vi "fgv_viLauch.vi"(7 "Option":T1(ring), 8 "Error In":errorcluster, 10 "vi path":path, 11 "UI in":refnum<class "UI.lvclass">) -> (0 "Error Out":errorcluster, 2 "VI ref Out":refnum<vi>, 3 "UI out":refnum<class "UI.lvclass">)   [LabVIEW 2018, in "Panel.lvclass"]
uses:
  Panel.lvclass
  User Interface/UI.lvclass
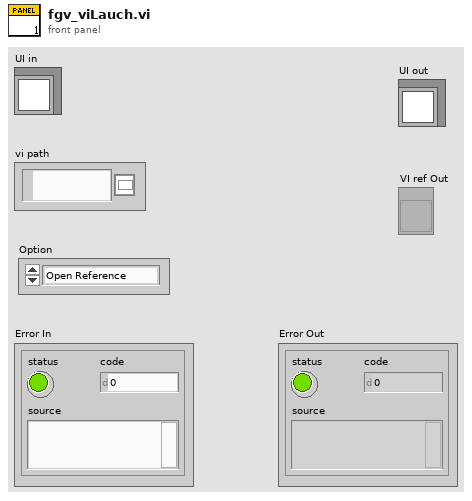
[diagram p1: front panel]
types:
  T1 = enum16{"Open Reference", "Launch VI", "Get VI Outputs"}
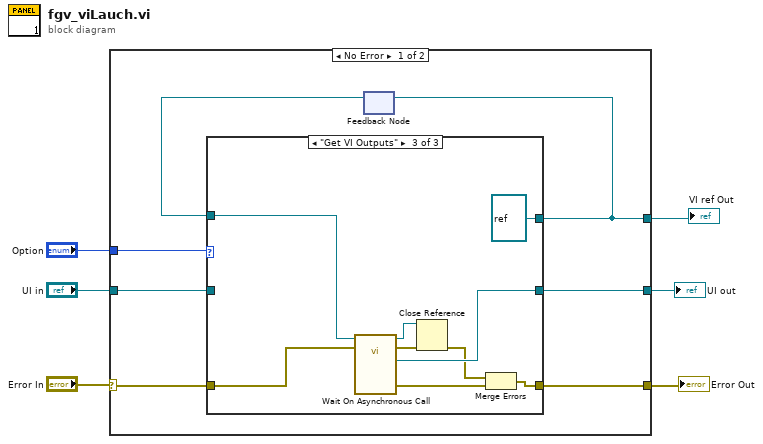
[diagram p0: block diagram]
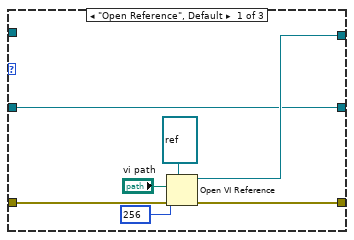
[diagram p2: hidden frame]
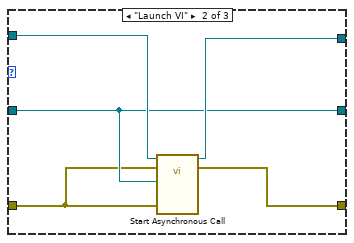
[diagram p3: hidden frame]
diagram:
  n1 = case shown="No Error" "Error In" {
    selector: "Error In" -> [w13 w35]
    tunnel: [w12 w35] -> w5
    tunnel: "Option" -> [w11 _]
    tunnel: [w9 w36] -> w3
    tunnel: "UI in" -> [w8 w36]
    tunnel: [w7 _] -> w1
    frame No Error {
      n2 = feedback #1() -> (w10:refnum<vi>)  [unwired: 1 in]
      n3 = case shown="\"Get VI Outputs\"" w11 {
        tunnel: w13 -> [w20 w21 w34]
        tunnel: [w19 w25 w30] -> w12
        tunnel: w10 -> [_ w24 w32]
        tunnel: [w18 w23 refnum<vi> refnum ("type specifier VI Refnum (for type only)")] -> w7
        tunnel: [w16 w22 w31] -> w9
        tunnel: w8 -> [w16 w22 _]
        frame "Open Reference", Default {
          n4 = Open VI Reference(type specifier VI Refnum (for type only)=refnum<vi> refnum, vi path="vi path", options=256, error in (no error)=w20) -> (vi reference=w18:refnum<vi>, error out=w19:errorcluster)  [unwired: 2 in]
        }
        frame "Launch VI" {
          n5 = call-by-ref "Start Asynchronous Call"(reference=w24, error in=w21, 8:"error in (no error)"=w21, "UI in"=w22) -> (reference out=w23:refnum<vi>, error out=w25:errorcluster)  [unwired: 8 in, 2 out]
        }
        frame "Get VI Outputs" {
          n6 = call-by-ref "Wait On Asynchronous Call"(reference=w32, error in=w34) -> (reference out=w27:refnum<vi>, error out=w33:errorcluster, 0:"error out"=w29:errorcluster, "UI out"=w31:refnum<class "UI.lvclass">)  [unwired: 10 in]
          n7 = Close Reference(reference=w27, error in (no error)=w33) -> (error out=w28:errorcluster)
          n8 = Merge Errors(w28, w29) -> (w30:errorcluster)
        }
      }
      n9 = feedback-in #1(w7) -> ()
    }
    frame Error {
    }
  }
  "Error Out" <- w5
  "UI out" <- w3
  "VI ref Out" <- w1
